vi "Alligent_DrawOverLay.vi"(10 "Image":T1) -> (0 "Y/2":dbl, 1 "X/2":dbl, 2 "Image Out":T1)   [LabVIEW 2018]
uses:
  <vilib>/vision/Image Controls.llb/IMAQ Image.ctl
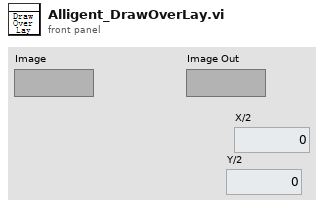
[diagram p1: front panel]
types:
  T1 = typedef "IMAQ Image.ctl" = refnum<image>
  T2 = cluster{"Left":i32, "Top":i32, "Right":i32, "Bottom":i32}
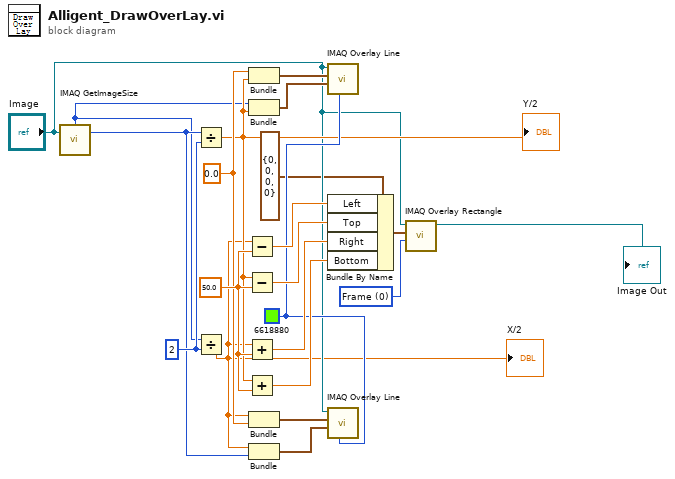
[diagram p0: block diagram]
diagram:
  w8 = u32 6618880 ("Color")
  w7 = 0.0
  w14 = u32 0 items=["Frame", "Fill", "Highlight"] ("Drawing Mode (Frame)")
  w17 = 50.0 ("y")
  w21 = 2 ("y")
  n1 = call "IMAQ GetImageSize"("Image"="Image") -> ("Y Resolution"=w13:i32, "X Resolution"=w5:i32)  [unwired: 3 in, 1 out]
  n2 = Divide(x=w13, y=w21) -> (x/y=w6:dbl)
  "Y/2" <- w6
  n3 = Divide(x=w5, y=w21) -> (x/y=w1:dbl)
  "X/2" <- w1
  n4 = Subtract(x=w1, y=w17) -> (x-y=w20:dbl)
  n5 = Subtract(x=w6, y=w17) -> (x-y=w19:dbl)
  n6 = Add(x=w1, y=w17) -> (x+y=w18:dbl)
  n7 = Add(x=w6, y=w17) -> (x+y=w16:dbl)
  n8 = Bundle(w7, w6) -> (w10:cluster{dbl, dbl})  [unwired: 1 in]
  n9 = Bundle("X Resolution"=w5, w6) -> (w9:cluster{"X Resolution":i32, dbl})  [unwired: 1 in]
  n10 = Bundle(w1, w7) -> (w12:cluster{dbl, dbl})  [unwired: 1 in]
  n11 = Bundle(w1, "Y Resolution"=w13) -> (w11:cluster{dbl, "Y Resolution":i32})  [unwired: 1 in]
  n12 = call "IMAQ Overlay Line"("Color"=w8, "End Point"=w9, "Start Point"=w10, "Image"="Image") -> ()  [unwired: 6 in, 2 out]
  n13 = Bundle By Name(cluster=T2 {"Left"=0, "Top"=0, "Right"=0, "Bottom"=0} ("Rectangle"), "Left"=w20, "Top"=w19, "Right"=w18, "Bottom"=w16) -> (w15:T2)
  n14 = call "IMAQ Overlay Line"("Color"=w8, "End Point"=w11, "Start Point"=w12, "Image"="Image") -> ()  [unwired: 6 in, 2 out]
  n15 = call "IMAQ Overlay Rectangle"("Drawing Mode (Frame)"=w14, "Rectangle"=w15, "Image"="Image") -> ("Image Out"=→"Image Out":T1)  [unwired: 7 in, 1 out]
